vi "LM Two T-Connected Gaussians and gradient.vi"(3 "output control":T1, 4 "data":variant, 5 "X":dbl[](array[numeric]), 6 "a":dbl[](array[numeric])) -> (0 "error out":errorcluster, 1 "f'(X,a)":dbl[][](array[numeric]), 2 "f(X,a)":dbl[](array[numeric]))   [LabVIEW 2021, in "Fits.lvlib"]
doc: "This template is the starting point for creating a model function to be passed to the Nonlinear Curve Fit.vi."
uses:
  Fits.lvlib
  <vilib>/gmath/NumericalOptimization/LM_output select.ctl
  D-Only Fixed Parameters.ctl
  <vilib>/gmath/NI_Gmath.lvlib
panel:
  # "Parameters:\n\nAmplitude 1: A1\nCenter 1: t1\nSDV 1: s1\nAmplitude 2: A2\nCenter 2: t2\nSDV 2: s2\n\nBridge Amplitude: A3 (or b)\nBridge Slope: a"
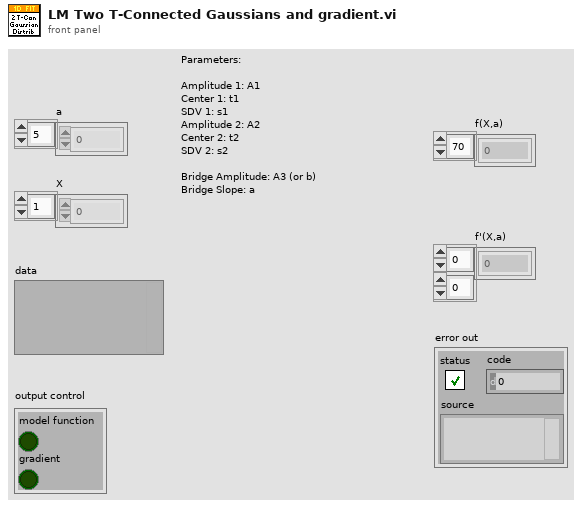
[diagram p1: front panel]
types:
  T1 = typedef "NI_Gmath.lvlib/LM_output select.ctl" = cluster{"model function":bool, "gradient":bool}
  T2 = typedef "Fits.lvlib/D-Only Fixed Parameters.ctl" = cluster{"Fix D-only Peak Location":bool, "Peak Location":dbl, "Fix D-only Peak FWHM":bool, "Peak FWHM":dbl}
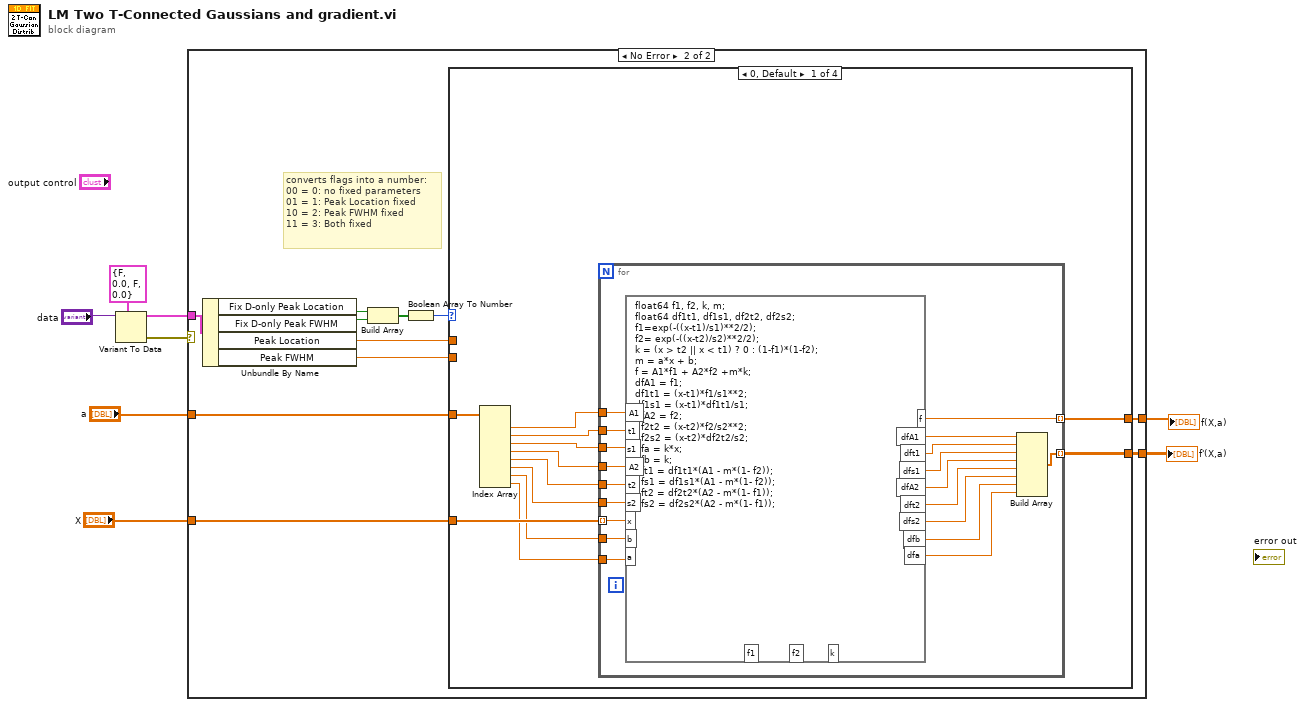
[diagram p0: block diagram]
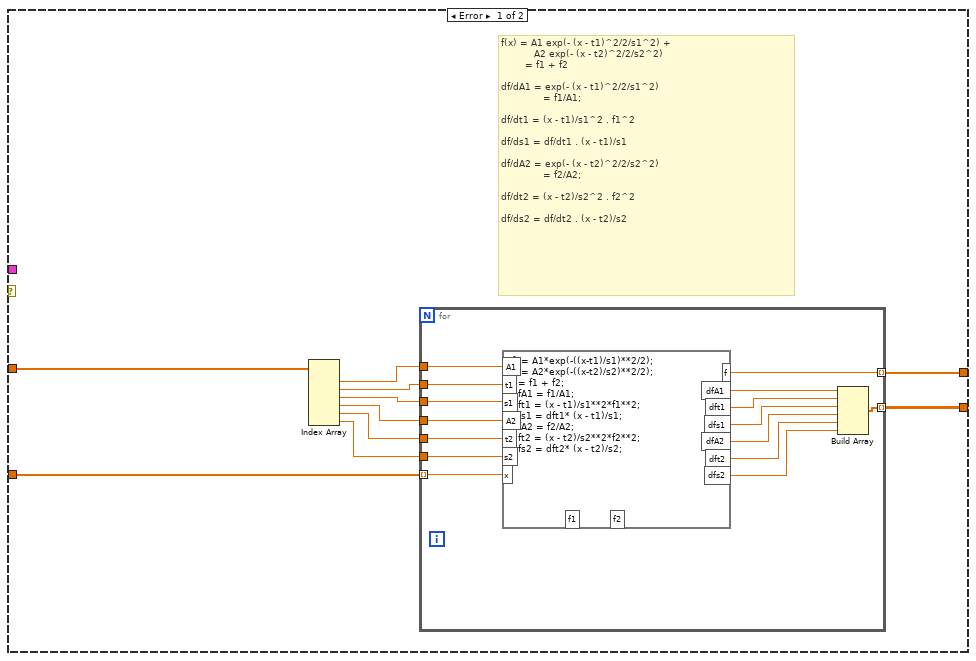
[diagram p2: hidden frame]
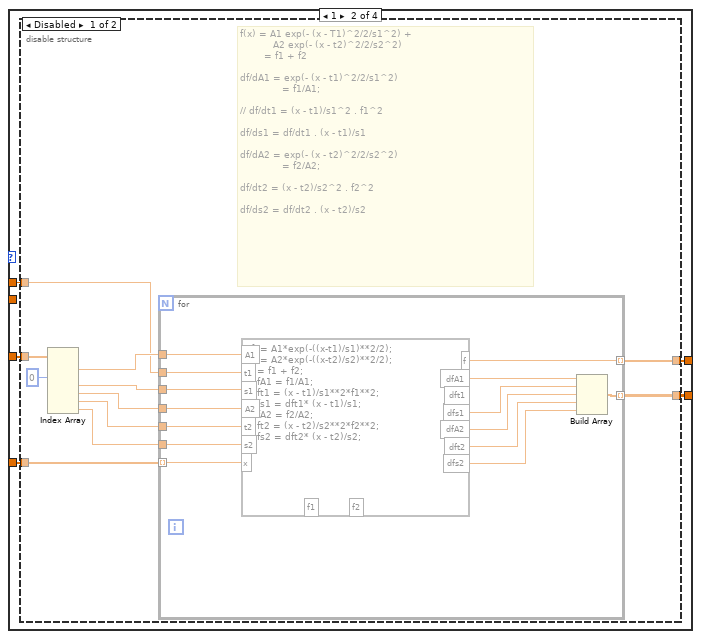
[diagram p3: hidden frame]
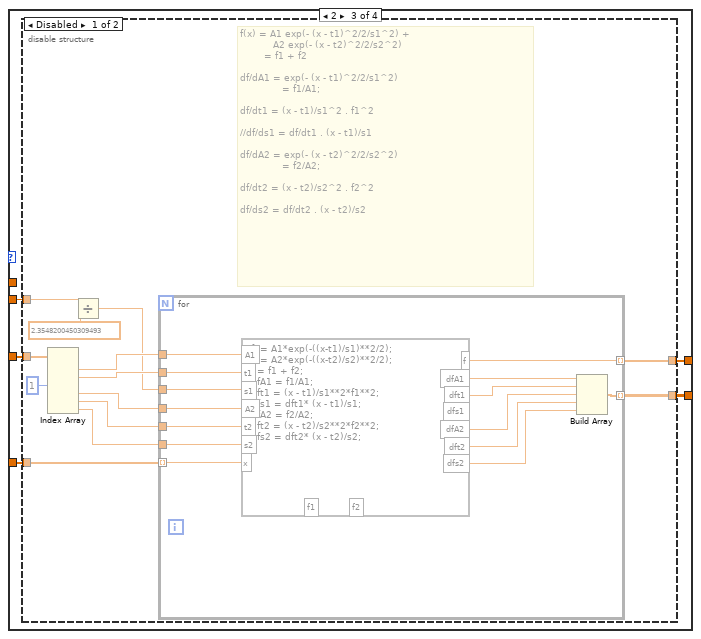
[diagram p5: hidden frame]
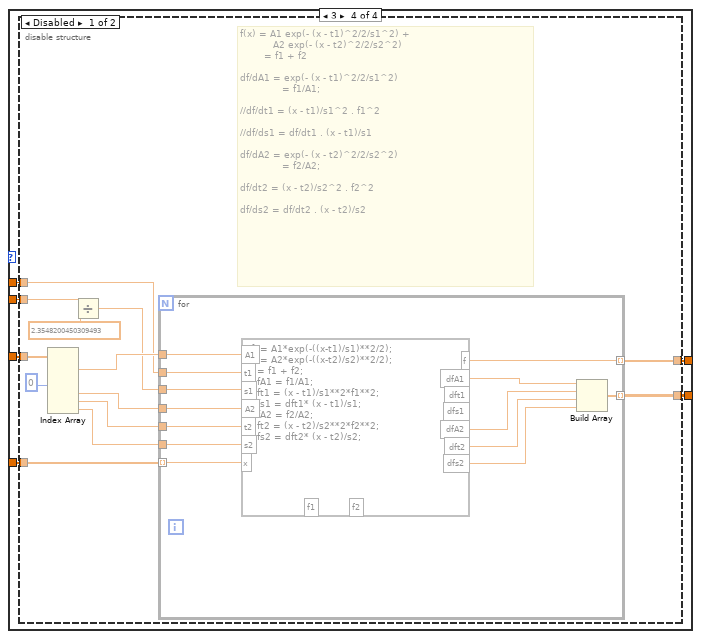
[diagram p7: hidden frame]
diagram:
  n1 = Variant To Data(type=T2 {"Fix D-only Peak Location"=FALSE, "Peak Location"=0.0, "Fix D-only Peak FWHM"=FALSE, "Peak FWHM"=0.0} ("Fixed Parameters"), Variant="data") -> (data=w1:T2, error out=w2:errorcluster)  [unwired: 1 in]
  n2 = case shown="No Error" w2 {
    tunnel: "a" -> [w18 w44]
    tunnel: "X" -> [w17 w43]
    tunnel: [w16 w42] -> w6
    tunnel: [w15 w41] -> w5
    tunnel: w1 -> [_ w40]
    frame Error {
      # "f(x) = A1 exp(- (x - t1)^2/2/s1^2) +\n           A2 exp(- (x - t2)^2/2/s2^2)\n        = f1 + f2\n\ndf/dA1 = exp(- (x - t1)^2/2/s1^2)\n              = f1/A1;\n\ndf/dt1 = (x - t1)/s1^2 . f1^2\n\ndf/ds1 = df/dt1 . (x - t1)/s1                     \n\ndf/dA2 = exp(- (x - t2)^2/2/s2^2)\n              = f2/A2;\n\ndf/dt2 = (x - t2)/s2^2 . f2^2\n\ndf/ds2 = df/dt2 . (x - t2)/s2"
      n3 = Index Array(array=w18) -> (element #1=w14:dbl, element #2=w13:dbl, element #3=w12:dbl, element #4=w11:dbl, element #5=w10:dbl, element #6=w9:dbl)  [unwired: 6 in]
      n4 = for {
        tunnel: w17 -> [w33] mode=indexing
        tunnel: [w31] -> w16 mode=indexing
        tunnel: [w30] -> w15 mode=indexing
        tunnel: w14 -> [w29]
        tunnel: w13 -> [w28]
        tunnel: w12 -> [w27]
        tunnel: w11 -> [w26]
        tunnel: w10 -> [w25]
        tunnel: w9 -> [w24]
        n5 = formula code="f1= A1*exp(-((x-t1)/s1)**2/2);\nf2= A2*exp(-((x-t2)/s2)**2/2);\nf = f1 + f2;\ndfA1 = f1/A1;\ndft1 = (x - t1)/s1**2*f1**2;\ndfs1 = dft1* (x - t1)/s1;\ndfA2 = f2/A2;\ndft2 = (x - t2)/s2**2*f2**2;\ndfs2 = dft2* (x - t2)/s2;"("A1"=w29, "t1"=w28, "s1"=w27, "x"=w33, "A2"=w26, "t2"=w25, "s2"=w24) -> ("f"=w31:dbl, "dfA1"=w32:dbl, "dft1"=w23:dbl, "dfs1"=w22:dbl, "dfA2"=w21:dbl, "dft2"=w20:dbl, "dfs2"=w19:dbl)  [unwired: 2 out]
        n6 = Build Array(w32, w23, w22, w21, w20, w19) -> (w30:dbl[])
      }
    }
    frame No Error {
      # "converts flags into a number:\n00 = 0: no fixed parameters\n01 = 1: Peak Location fixed\n10 = 2: Peak FWHM fixed\n11 = 3: Both fixed"
      n7 = Unbundle By Name(w40) -> ("Fix D-only Peak Location"=w39:bool, "Fix D-only Peak FWHM"=w38:bool, "Peak Location"=w35:dbl, "Peak FWHM"=w34:dbl)
      n8 = Build Array(w39, w38) -> (w37:bool[])
      n9 = Boolean Array To Number(Boolean array=w37) -> (number=w36:u32)
      n10 = case shown="0, Default" w36 {
        tunnel: w44 -> [w56 w80 w110 w143]
        tunnel: w43 -> [w55 w79 w109 w142]
        tunnel: [w54 w78 w108 w141] -> w42
        tunnel: [w53 w77 w107 w140] -> w41
        tunnel: w35 -> [_ w76 _ w138]
        tunnel: w34 -> [_ _ w106 w139]
        frame 0, Default {
          n11 = Index Array(array=w56) -> (element #1=w52:dbl, element #2=w51:dbl, element #3=w50:dbl, element #4=w49:dbl, element #5=w48:dbl, element #6=w47:dbl, element #7=w46:dbl, element #8=w45:dbl)  [unwired: 8 in]
          n12 = for {
            tunnel: w55 -> [w75] mode=indexing
            tunnel: [w73] -> w54 mode=indexing
            tunnel: [w72] -> w53 mode=indexing
            tunnel: w52 -> [w71]
            tunnel: w51 -> [w70]
            tunnel: w50 -> [w69]
            tunnel: w49 -> [w68]
            tunnel: w48 -> [w67]
            tunnel: w47 -> [w66]
            tunnel: w46 -> [w60]
            tunnel: w45 -> [w58]
            n13 = formula code="float64 f1, f2, k, m;\nfloat64 df1t1, df1s1, df2t2, df2s2;\nf1=exp(-((x-t1)/s1)**2/2);\nf2= exp(-((x-t2)/s2)**2/2);\nk = (x > t2 || x < t1) ? 0 : (1-f1)*(1-f2);\nm = a*x + b;\nf = A1*f1 + A2*f2 +m*k;\ndfA1 = f1;\ndf1t1 = (x-t1)*f1/s1**2;\ndf1s1 = (x-t1)*df1t1/s1;\ndfA2 = f2;\ndf2t2 = (x-t2)*f2/s2**2;\ndf2s2 = (x-t2)*df2t2/s2;\ndfa = k*x;\ndfb = k;\ndft1 = df1t1*(A1 - m*(1- f2));\ndfs1 = df1s1*(A1 - m*(1- f2));\ndft2 = df2t2*(A2 - m*(1- f1));\ndfs2 = df2s2*(A2 - m*(1- f1));"("A1"=w71, "t1"=w70, "s1"=w69, "x"=w75, "A2"=w68, "t2"=w67, "s2"=w66, "b"=w60, "a"=w58) -> ("f"=w73:dbl, "dfA1"=w74:dbl, "dft1"=w65:dbl, "dfs1"=w64:dbl, "dfA2"=w63:dbl, "dft2"=w62:dbl, "dfs2"=w61:dbl, "dfb"=w59:dbl, "dfa"=w57:dbl)  [unwired: 3 out]
            n14 = Build Array(w74, w65, w64, w63, w62, w61, w59, w57) -> (w72:dbl[])
          }
        }
        frame 1 {
          n15 = disable-structure shown="Disabled" {
            disable-tunnel: w80 -> [w91 _]
            disable-tunnel: w79 -> [w90 _]
            disable-tunnel: [w89 _] -> w78
            disable-tunnel: [w88 _] -> w77
            disable-tunnel: w76 -> [w82 _]
            frame Disabled {
              # "f(x) = A1 exp(- (x - T1)^2/2/s1^2) +\n           A2 exp(- (x - t2)^2/2/s2^2)\n        = f1 + f2\n\ndf/dA1 = exp(- (x - t1)^2/2/s1^2)\n              = f1/A1;\n\n// df/dt1 = (x - t1)/s1^2 . f1^2\n\ndf/ds1 = df/dt1 . (x - t1)/s1                     \n\ndf/dA2 = exp(- (x - t2)^2/2/s2^2)\n              = f2/A2;\n\ndf/dt2 = (x - t2)/s2^2 . f2^2\n\ndf/ds2 = df/dt2 . (x - t2)/s2"
              n16 = Index Array(array=w91, index #2=0 ("index")) -> (element #1=w87:dbl, element #3=w86:dbl, element #4=w85:dbl, element #5=w84:dbl, element #6=w83:dbl)  [unwired: 5 in, 1 out]
              n17 = for {
                tunnel: w90 -> [w105] mode=indexing
                tunnel: [w103] -> w89 mode=indexing
                tunnel: [w102] -> w88 mode=indexing
                tunnel: w87 -> [w101]
                tunnel: w82 -> [w100]
                tunnel: w86 -> [w99]
                tunnel: w85 -> [w98]
                tunnel: w84 -> [w97]
                tunnel: w83 -> [w96]
                n18 = formula code="f1= A1*exp(-((x-t1)/s1)**2/2);\nf2= A2*exp(-((x-t2)/s2)**2/2);\nf = f1 + f2;\ndfA1 = f1/A1;\ndft1 = (x - t1)/s1**2*f1**2;\ndfs1 = dft1* (x - t1)/s1;\ndfA2 = f2/A2;\ndft2 = (x - t2)/s2**2*f2**2;\ndfs2 = dft2* (x - t2)/s2;"("A1"=w101, "t1"=w100, "s1"=w99, "x"=w105, "A2"=w98, "t2"=w97, "s2"=w96) -> ("f"=w103:dbl, "dfA1"=w104:dbl, "dfs1"=w95:dbl, "dfA2"=w94:dbl, "dft2"=w93:dbl, "dfs2"=w92:dbl)  [unwired: 3 out]
                n19 = Build Array(w104, w95, w94, w93, w92) -> (w102:dbl[])
              }
            }
            frame Enabled {
            }
          }
        }
        frame 2 {
          n20 = disable-structure shown="Disabled" {
            disable-tunnel: w110 -> [w123 _]
            disable-tunnel: w109 -> [w122 _]
            disable-tunnel: [w121 _] -> w108
            disable-tunnel: [w120 _] -> w107
            disable-tunnel: w106 -> [w114 _]
            frame Disabled {
              # "f(x) = A1 exp(- (x - t1)^2/2/s1^2) +\n           A2 exp(- (x - t2)^2/2/s2^2)\n        = f1 + f2\n\ndf/dA1 = exp(- (x - t1)^2/2/s1^2)\n              = f1/A1;\n\ndf/dt1 = (x - t1)/s1^2 . f1^2\n\n//df/ds1 = df/dt1 . (x - t1)/s1                     \n\ndf/dA2 = exp(- (x - t2)^2/2/s2^2)\n              = f2/A2;\n\ndf/dt2 = (x - t2)/s2^2 . f2^2\n\ndf/ds2 = df/dt2 . (x - t2)/s2"
              n21 = Index Array(array=w123, index #3=1 ("index")) -> (element #1=w119:dbl, element #2=w118:dbl, element #4=w117:dbl, element #5=w116:dbl, element #6=w115:dbl)  [unwired: 5 in, 1 out]
              n22 = Divide(x=w114, y=2.3548200450309493) -> (x/y=w112:dbl)
              n23 = for {
                tunnel: w122 -> [w137] mode=indexing
                tunnel: [w135] -> w121 mode=indexing
                tunnel: [w134] -> w120 mode=indexing
                tunnel: w119 -> [w133]
                tunnel: w118 -> [w132]
                tunnel: w112 -> [w131]
                tunnel: w117 -> [w130]
                tunnel: w116 -> [w129]
                tunnel: w115 -> [w128]
                n24 = formula code="f1= A1*exp(-((x-t1)/s1)**2/2);\nf2= A2*exp(-((x-t2)/s2)**2/2);\nf = f1 + f2;\ndfA1 = f1/A1;\ndft1 = (x - t1)/s1**2*f1**2;\ndfs1 = dft1* (x - t1)/s1;\ndfA2 = f2/A2;\ndft2 = (x - t2)/s2**2*f2**2;\ndfs2 = dft2* (x - t2)/s2;"("A1"=w133, "t1"=w132, "s1"=w131, "x"=w137, "A2"=w130, "t2"=w129, "s2"=w128) -> ("f"=w135:dbl, "dfA1"=w136:dbl, "dft1"=w127:dbl, "dfA2"=w126:dbl, "dft2"=w125:dbl, "dfs2"=w124:dbl)  [unwired: 3 out]
                n25 = Build Array(w136, w127, w126, w125, w124) -> (w134:dbl[])
              }
            }
            frame Enabled {
            }
          }
        }
        frame 3 {
          n26 = disable-structure shown="Disabled" {
            disable-tunnel: w143 -> [w156 _]
            disable-tunnel: w142 -> [w155 _]
            disable-tunnel: [w154 _] -> w141
            disable-tunnel: [w153 _] -> w140
            disable-tunnel: w139 -> [w148 _]
            disable-tunnel: w138 -> [w145 _]
            frame Disabled {
              # "f(x) = A1 exp(- (x - t1)^2/2/s1^2) +\n           A2 exp(- (x - t2)^2/2/s2^2)\n        = f1 + f2\n\ndf/dA1 = exp(- (x - t1)^2/2/s1^2)\n              = f1/A1;\n\n//df/dt1 = (x - t1)/s1^2 . f1^2\n\n//df/ds1 = df/dt1 . (x - t1)/s1                     \n\ndf/dA2 = exp(- (x - t2)^2/2/s2^2)\n              = f2/A2;\n\ndf/dt2 = (x - t2)/s2^2 . f2^2\n\ndf/ds2 = df/dt2 . (x - t2)/s2"
              n27 = Index Array(array=w156, index #3=0 ("index")) -> (element #1=w152:dbl, element #4=w151:dbl, element #5=w150:dbl, element #6=w149:dbl)  [unwired: 5 in, 2 out]
              n28 = Divide(x=w148, y=2.3548200450309493) -> (x/y=w146:dbl)
              n29 = for {
                tunnel: w155 -> [w169] mode=indexing
                tunnel: [w167] -> w154 mode=indexing
                tunnel: [w166] -> w153 mode=indexing
                tunnel: w152 -> [w165]
                tunnel: w145 -> [w164]
                tunnel: w146 -> [w163]
                tunnel: w151 -> [w162]
                tunnel: w150 -> [w161]
                tunnel: w149 -> [w160]
                n30 = formula code="f1= A1*exp(-((x-t1)/s1)**2/2);\nf2= A2*exp(-((x-t2)/s2)**2/2);\nf = f1 + f2;\ndfA1 = f1/A1;\ndft1 = (x - t1)/s1**2*f1**2;\ndfs1 = dft1* (x - t1)/s1;\ndfA2 = f2/A2;\ndft2 = (x - t2)/s2**2*f2**2;\ndfs2 = dft2* (x - t2)/s2;"("A1"=w165, "t1"=w164, "s1"=w163, "x"=w169, "A2"=w162, "t2"=w161, "s2"=w160) -> ("f"=w167:dbl, "dfA1"=w168:dbl, "dfA2"=w159:dbl, "dft2"=w158:dbl, "dfs2"=w157:dbl)  [unwired: 4 out]
                n31 = Build Array(w168, w159, w158, w157) -> (w166:dbl[])
              }
            }
            frame Enabled {
            }
          }
        }
      }
    }
  }
  "f(X,a)" <- w6
  "f'(X,a)" <- w5
